vi "main_remote_old.vi"() -> ()   [LabVIEW 2019]
uses:
  Ctrl/SoutWork.ctl
  <vilib>/Utility/inputDevices.llb/keyboardAcquire.vi
  <vilib>/Utility/inputDevices.llb/closeKeyboard.vi
panel:
  in  "AGV status":string
  in  "buttton group":T1
  in  "tap":T2(tab)
  out "LiDAR Image Gray":T3(plugin-control)
  out "LiDAR Error":errorcluster
  out "Robot Status Error":errorcluster
  out "System Status Error":errorcluster
  out "Remote Control Command Error":errorcluster
  out "Vehicle Motion State Error":errorcluster
  in  "EStop Command":bool
  in  "Manual":bool
  in  "ChoosePath":u8
  in  "Stop AGV":bool
  in  "AGV Start":bool
  out "Error code high":bool[](array[boolean])
  out "Error code  low":bool[](array[boolean])
  out "Motor Over Current Alarm":bool
  out "Motor Over Current Protection":bool
  out "Motor Drive Over Temperature":bool
  out "System Status":T4
  out "Vehicle Motion State":T5
  out "robot status":T6
  out "Sensor Status":T7
  out "EStop Pressed":bool
  out "Image":T3(plugin-control)
  in  "OnboardPC IP":string="223.171.56.43"
  out "Index Y":dbl
  out "Index X":dbl
  out "Translational Vel (m/s)":dbl format="%4.2f"
  out "Rotational Vel (rad/s)":dbl format="%.2f"
  in  "stop":bool
  # "Mando GOLIE"
  # "Communication Error"
  # "<E-H>\nbit [0] Check error of CAN communication control command (0: No failure 1: Failure) \nbit [1] Motor drive over-temperature alarm[1] (0: No alarm 1: Alarm) Temperature limited to 55℃ \nbit [2] Motor over-current alarm[1] (0: No alarm 1: Alarm) Current effective value 15A \nbit [3] Battery under-voltage alarm (0: No alarm 1: Alarm) Alarm voltage 22.5V \nbit [4] RC transmitter disconnection protection (0: Normal 1: RC transmitter disconnected) \n\n<E-L>\nbit [0] Battery under-voltage failure (0: No failure 1: Failure) Protective voltage 22V \nbit [1] Battery over-voltage failure (0: No failure 1: Failure)  \nbit [2] No.1 motor communication failure (0: No failure 1: Failure)  \nbit [3] No.2 motor communication failure (0: No failure 1: Failure)  \nbit [4] No.3 motor communication failure (0: No failure 1: Failure)  \nbit [5] No.4 motor communication failure (0: No failure 1: Failure)  \nbit [6] Motor drive over-temperature protection[2] (0: No protection 1: Protection) Temperature limited to 65℃ \nbit [7] Motor over-current protection[2] (0: No protection 1: Protection) Current effective value 20A"
  # "bit [0] Battery under-voltage failure (0: No failure 1: Failure) Protective voltage 22V \nbit [1] Battery over-voltage failure (0: No failure 1: Failure)  \nbit [2] No.1 motor communication failure (0: No failure 1: Failure)  \nbit [3] No.2 motor communication failure (0: No failure 1: Failure)  \nbit [4] No.3 motor communication failure (0: No failure 1: Failure)  \nbit [5] No.4 motor communication failure (0: No failure 1: Failure)  \nbit [6] Motor drive over-temperature protection[2] (0: No protection 1: Protection) Temperature limited to 65℃ \nbit [7] Motor over-current protection[2] (0: No protection 1: Protection) Current effective value 20A"
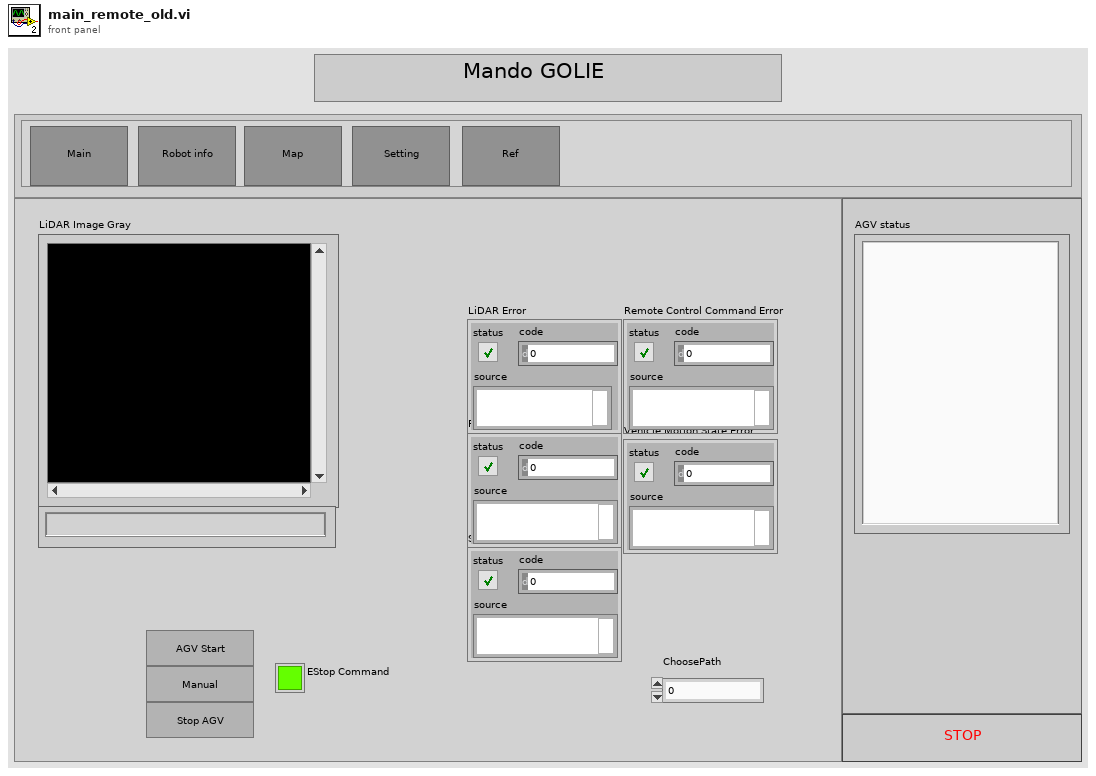
[diagram p1: front panel]
types:
  T1 = cluster{"Main":bool, "Main 2":bool, "Main 3":bool, "Main 4":bool, "Main 5":bool}
  T2 = enum32{"Main", "Robot info", "Map", "Setting", "Ref"}
  T3 = typedef "IMAQ Image.ctl" = refnum<image>
  T4 = cluster{"System Feedback":cluster{"system state":string, "Control Mode":u8, "Battery Voltage (V)":dbl, "error code High":u8, "error code Low":u8}}
  T5 = typedef "SoutWork.ctl" = enum16{"wait", "Move", "ObstacleStop", "EStop", "Goal"}
  T6 = cluster{"X (m)":dbl, "Y (m)":dbl, "Z (m)":dbl, "Roll (degree)":dbl, "Pitch (degree)":dbl, "Heading (degree)":dbl, "Linear velocity (m/s)":dbl, "Angular velocity (rad/s)":dbl}
  T7 = cluster{"VLP16 Sensor Error ":bool, "SICK Sensor Error":bool, "GNSS Sensor Error":bool, "Heading=0 Alarm":bool, "Obstacle Stop Alarm":bool}
  T8 = typedef "Image Type" = u32
  T9 = enum16{"0", "1", "2", "3", "4", "5", "6", "7", "8", "9", "A", "B", "C", "D", "E", "F", "G", "H", "I", "J", "K", "L", "M", "N", "O", "P", "Q", "R", "S", "T", "U", "V", "W", "X", "Y", "Z", "F1", "F2", "F3", "F4", "F5", "F6", "F7", "F8", "F9", "F10", "F11", "F12", "F13", "F14", "F15", "ADD", "BACK", "BACKSLASH", "CAPITAL", "COMMA", "DECIMAL", "DELETE", "DIVIDE", "DOWN", "END", "EQUALS", "ESCAPE", "GRAVE (`)", "HOME", "INSERT", "LBRACKET", "LCONTROL", "LEFT", "L ALT", "LSHIFT", "LWIN", "MINUS", "MULTIPLY", "NEXT", "NUMLOCK", "NUMPAD_0", "NUMPAD_1", "NUMPAD_2", "NUMPAD_3", "NUMPAD_4", "NUMPAD_5", "NUMPAD_6", "NUMPAD_7", "NUMPAD_8", "NUMPAD_9", "PAUSE", "PERIOD", "PRIOR (PG UP)", "RBRACKET", "RCONTROL", "RETURN", "RIGHT", "R ALT", "RSHIFT", "RWIN", "SCROLL", "SEMICOLON", "SLASH", "SPACE", "SUBTRACT", "TAB", "UP", "ENTER (num pad)", "' (quote)"}[]
  T10 = enum16{"0", "1", "2", "3", "4", "5", "6", "7", "8", "9", "A", "B", "C", "D", "E", "F", "G", "H", "I", "J", "K", "L", "M", "N", "O", "P", "Q", "R", "S", "T", "U", "V", "W", "X", "Y", "Z", "F1", "F2", "F3", "F4", "F5", "F6", "F7", "F8", "F9", "F10", "F11", "F12", "F13", "F14", "F15", "ADD", "BACK", "BACKSLASH", "CAPITAL", "COMMA", "DECIMAL", "DELETE", "DIVIDE", "DOWN", "END", "EQUALS", "ESCAPE", "GRAVE (`)", "HOME", "INSERT", "LBRACKET", "LCONTROL", "LEFT", "L ALT", "LSHIFT", "LWIN", "MINUS", "MULTIPLY", "NEXT", "NUMLOCK", "NUMPAD_0", "NUMPAD_1", "NUMPAD_2", "NUMPAD_3", "NUMPAD_4", "NUMPAD_5", "NUMPAD_6", "NUMPAD_7", "NUMPAD_8", "NUMPAD_9", "PAUSE", "PERIOD", "PRIOR (PG UP)", "RBRACKET", "RCONTROL", "RETURN", "RIGHT", "R ALT", "RSHIFT", "RWIN", "SCROLL", "SEMICOLON", "SLASH", "SPACE", "SUBTRACT", "TAB", "UP", "ENTER (num pad)", "' (quote)"}
  T11 = cluster{"Vehicle Motion State":u8, "Index X":dbl, "Index Y":dbl, bool}
  T12 = cluster{"Boolean array[0]":bool, "Boolean array[1]":bool, "Boolean array[2]":bool, "Boolean array[3]":bool, "Boolean array[4]":bool}
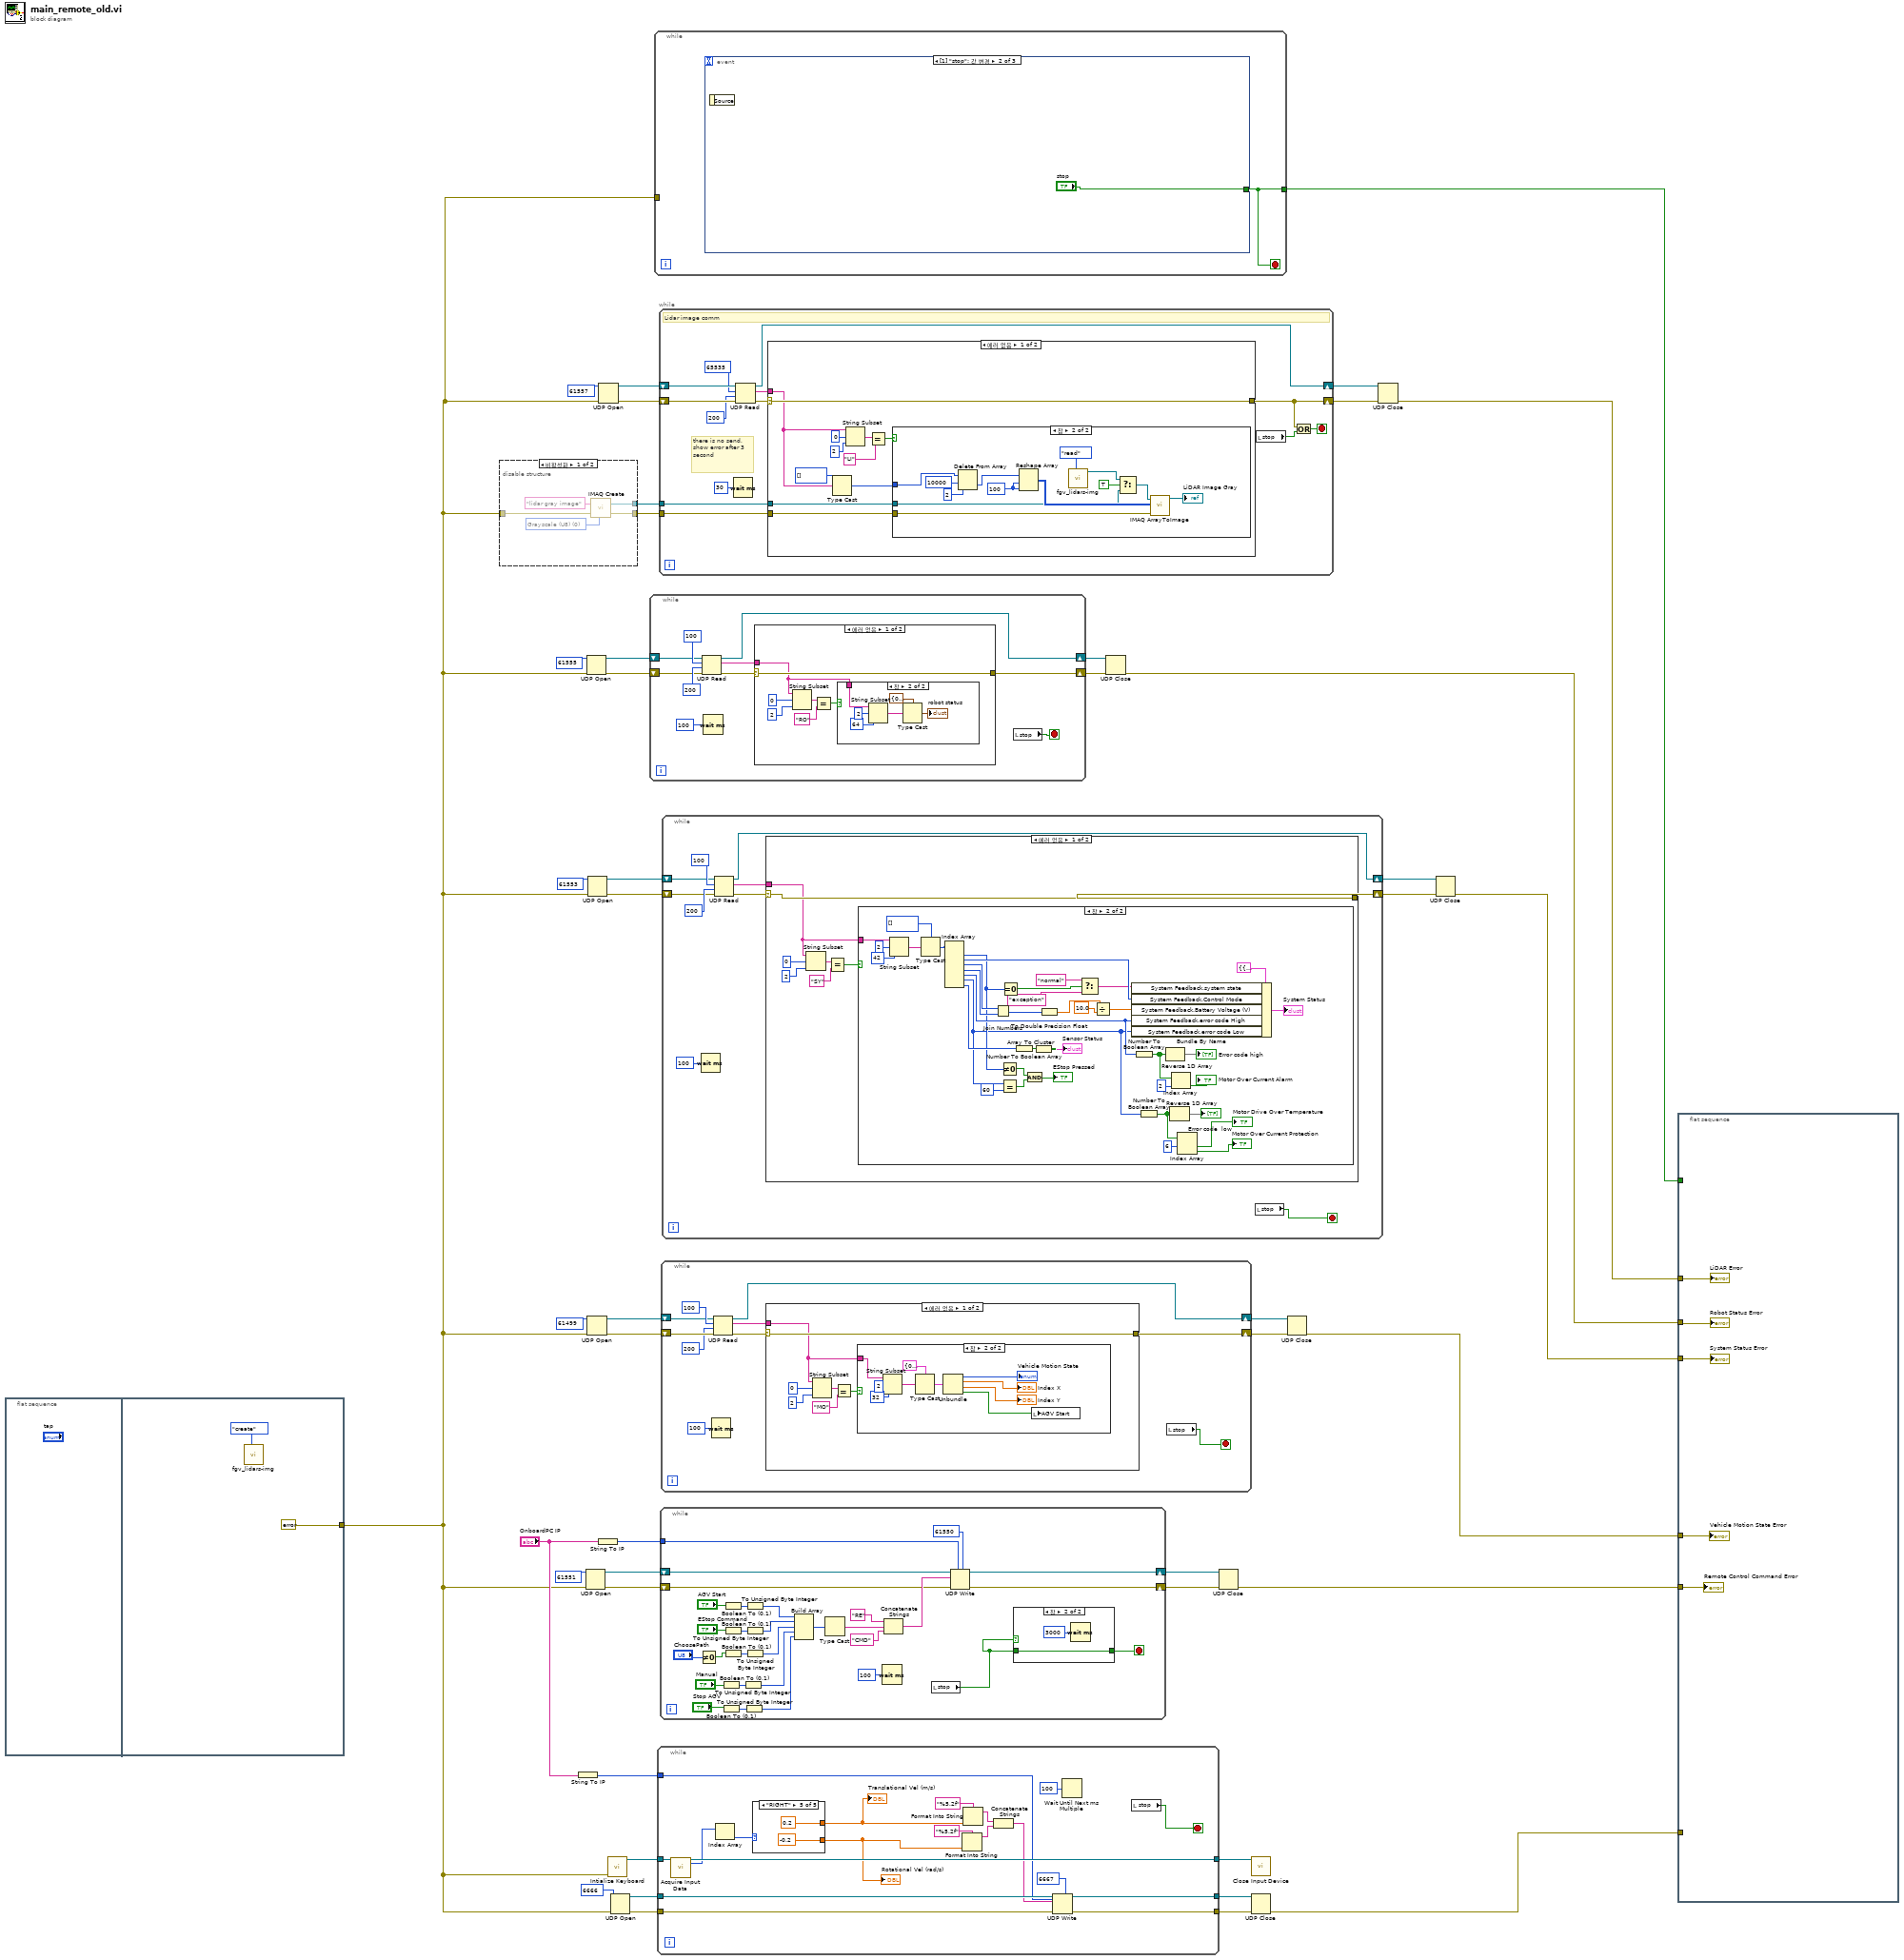
[diagram p0: block diagram]
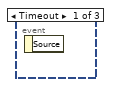
[diagram p3: hidden frame]
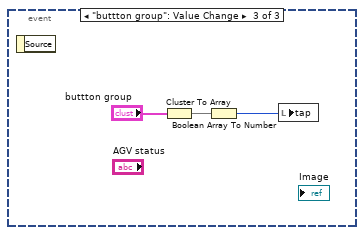
[diagram p4: hidden frame]
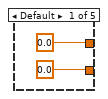
[diagram p5: hidden frame]
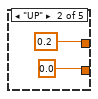
[diagram p6: hidden frame]
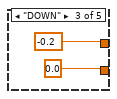
[diagram p7: hidden frame]
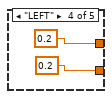
[diagram p8: hidden frame]
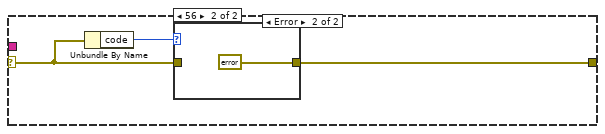
[diagram p10: hidden frame]
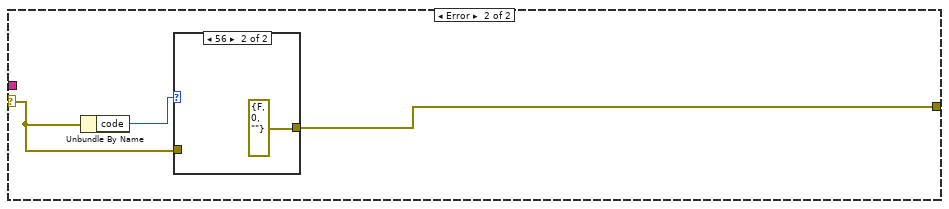
[diagram p14: hidden frame]
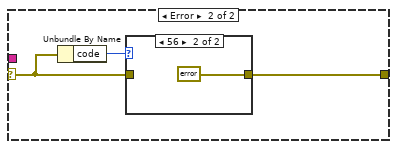
[diagram p17: hidden frame]
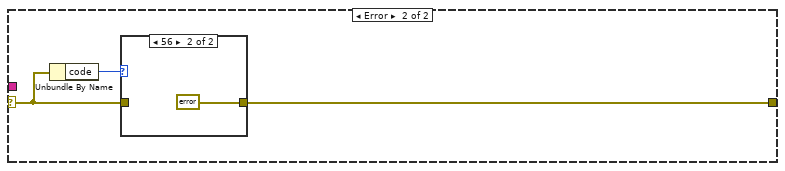
[diagram p20: hidden frame]
diagram:
  n1 = flat-sequence {
    tunnel: [errorcluster {"status"=FALSE, "code"=0, "source"=""} ("에러 입력(에러 없음)")] -> w8
    frame #0 {
    }
    frame #1 {
      n2 = call "fgv_lidars-img.vi"("cmd"=enum16{"create", "read", "close"}."create") -> ()  [unwired: 10 in, 1 out]
    }
  }
  n3 = disable-structure shown="비활성화" {
    disable-tunnel: [w50 _] -> w40
    disable-tunnel: [w49 _] -> w39
    disable-tunnel: w8 -> [w48 _]
    frame Disabled {
      w51 = T8 0 items=["Grayscale (U8)", "Grayscale (I16)", "Grayscale (SGL)", "Complex (CSG)", "RGB (U32)", "HSL (U32)", "RGB (U64)", "Grayscale (U16)"] ("Image Type")
      n4 = call "IMAQ Create"("Image Name"="lidar gray image", "Image Type"=w51, "error in (no error)"=w48) -> ("New Image"=w50:T3, "error out"=w49:errorcluster)  [unwired: 2 in]
    }
    frame Enabled {
    }
  }
  n5 = String To IP(1:"OnboardPC IP") -> (0:w9:u32)
  n6 = UDP Open(8:w8, 11:u16 61551 ("port")) -> (port=w27:refnum<k16>, 0:w26:errorcluster)  [unwired: 3 in, 1 out]
  n7 = UDP Open(8:w8, 11:u16 61555 ("port")) -> (port=w37:refnum<k16>, 0:w36:errorcluster)  [unwired: 3 in, 1 out]
  n8 = UDP Open(8:w8, 11:u16 61499 ("port")) -> (port=w21:refnum<k16>, 0:w20:errorcluster)  [unwired: 3 in, 1 out]
  n9 = UDP Open(8:w8, 11:u16 61553 ("port")) -> (port=w32:refnum<k16>, 0:w31:errorcluster)  [unwired: 3 in, 1 out]
  n10 = String To IP(1:"OnboardPC IP") -> (0:w23:u32)
  n11 = UDP Open(8:w8, 11:u16 61557 ("port")) -> (port=w45:refnum<k16>, 0:w44:errorcluster)  [unwired: 3 in, 1 out]
  n12 = call <vilib>:"Intialize Keyboard.vi"("error in (no error)"=w8) -> ("device ID"=w14:refnum<k1>)  [unwired: 9 in, 1 out]
  n13 = UDP Open(8:w8, 11:u16 6666 ("remote port or service name")) -> (port=w16:refnum<k16>, 0:w15:errorcluster)  [unwired: 3 in, 1 out]
  n14 = while {
    shift-right: [w56] -> w35
    shift-left: w37 -> [w60]
    shift-right: [w55] -> w34
    shift-left: w36 -> [w59]
    stop <- w53 stop-if-true
    n15 = UDP Read(connection ID=w60, max size (548)=100, timeout ms (25000)=200, 8:w59) -> (data out=w57:string, error out=w58:errorcluster, 3:w56:refnum<k16>)  [unwired: 2 out]
    n16 = Wait (ms)(milliseconds to wait=u32 100) -> ()  [unwired: 1 out]
    n17 = case shown="에러 없음" w58 {
      selector: w58 -> [w69 w77]
      tunnel: w57 -> [w63 _]
      tunnel: [w69 w76] -> w55
      frame No Error {
        n18 = String Subset(string=w63, offset (0)=0, length (rest)=2 ("length (rest)")) -> (substring=w66:string)
        n19 = Equal?(x=w66, y="RO") -> (x = y?=w64:bool)
        n20 = case shown="참" w64 {
          tunnel: w63 -> [_ w75]
          frame False {
          }
          frame True {
            n21 = String Subset(string=w75, offset (0)=2, length (rest)=64 ("length (rest)")) -> (substring=w71:string)
            n22 = Type Cast(type=T6 {"X (m)"=0.0, "Y (m)"=0.0, "Z (m)"=0.0, "Roll (degree)"=0.0, "Pitch (degree)"=0.0, "Heading (degree)"=0.0, "Linear velocity (m/s)"=0.0, "Angular velocity (rad/s)"=0.0} ("Robot Status"), x=w71) -> (*(type *) &x=→"robot status":T6)
          }
        }
      }
      frame Error {
        n23 = Unbundle By Name(w77) -> ("code"=w78:i32)
        n24 = case shown="56" w78 {
          tunnel: w77 -> [w79 _]
          tunnel: [w79 errorcluster {"status"=FALSE, "code"=0, "source"=""} ("error IO")] -> w76
          frame 0, Default {
          }
          frame 56 {
          }
        }
      }
    }
    n25 = local read "stop"() -> (w53:bool)
  }
  n26 = while {
    tunnel: w8 -> [_]
    tunnel: [w81] -> w1
    stop <- w81 stop-if-true
    n27 = event shown="[1] \"stop\": 값 변경" {
      selector: _ -> [_ _ _]
      dyn-events: _ -> [_ _ _]
      timeout: _ -> [_ _ _]
      tunnel: [_ "stop" _] -> w81
      event Timeout {
        n28 = event-data() -> ()  [unwired: 1 in, 1 out]
      }
      event "stop": Value Change {
        n29 = event-data() -> ()  [unwired: 1 in, 1 out]
      }
      event "buttton group": Value Change {
        n30 = event-data() -> ()  [unwired: 1 in, 1 out]
        n31 = Cluster To Array(cluster="buttton group") -> (array=w84:bool[])
        n32 = Boolean Array To Number(Boolean array=w84) -> (number=w83:u32)
        n33 = local write "tap"(w83) -> ()
      }
    }
  }
  n34 = while {
    tunnel: w14 -> [w104]
    tunnel: [w103] -> w17
    tunnel: w16 -> [w102]
    tunnel: [w101] -> w13
    tunnel: [w95] -> w12
    tunnel: w15 -> [w94]
    tunnel: w9 -> [w88]
    stop <- w86 stop-if-true
    # "Main Loop"
    n35 = call-poly <vilib>:"Acquire Input Data.vi"("device ID"=w104) -> ("device ID"=w103:refnum<k1>, "keys pressed"=w92:T9)  [unwired: 16 in, 1 out]
    n36 = Index Array(array=w92) -> (element=w91:T10)  [unwired: 1 in]
    n37 = case shown="\"RIGHT\"" w91 {
      tunnel: [0.0 ("Rotational Vel (rad/s)") 0.2 ("Rotational Vel (rad/s)") -0.2 ("Rotational Vel (rad/s)") 0.2 ("Rotational Vel (rad/s)") 0.2 ("Rotational Vel (rad/s)")] -> w90
      tunnel: [0.0 ("Rotational Vel (rad/s)") 0.0 ("Rotational Vel (rad/s)") 0.0 ("Rotational Vel (rad/s)") 0.2 ("Rotational Vel (rad/s)") -0.2 ("Rotational Vel (rad/s)")] -> w89
      frame Default {
      }
      frame "UP" {
      }
      frame "DOWN" {
      }
      frame "LEFT" {
      }
      frame "RIGHT" {
      }
    }
    "Translational Vel (m/s)" <- w90
    "Rotational Vel (rad/s)" <- w89
    n38 = Format Into String(format string="%5.2f", w89) -> (resulting string=w97:string)  [unwired: 2 in, 1 out]
    n39 = Format Into String(format string="%5.2f", w90) -> (resulting string=w98:string)  [unwired: 2 in, 1 out]
    n40 = Concatenate Strings(w98, w97) -> (w96:string)
    n41 = UDP Write(address=w88, port or service name=u16 6667, connection ID=w102, data in=w96, 8:w94) -> (error out=w95:errorcluster, 3:w101:refnum<k16>)  [unwired: 1 in]
    n42 = Wait Until Next ms Multiple(millisecond multiple=u32 100) -> ()  [unwired: 1 out]
    n43 = local read "stop"() -> (w86:bool)
  }
  n44 = while {
    shift-right: [w120] -> w43
    shift-left: w45 -> [w127]
    shift-right: [w119] -> w42
    shift-left: w44 -> [w126]
    tunnel: w40 -> [w118]
    tunnel: w39 -> [w117]
    stop <- w123 stop-if-true
    # "there is no send, show error after 3 second"
    # "Lidar image comm"
    n45 = Wait (ms)(milliseconds to wait=u32 30) -> ()  [unwired: 1 out]
    n46 = UDP Read(connection ID=w127, max size (548)=65535, timeout ms (25000)=200, 8:w126) -> (data out=w125:string, error out=w121:errorcluster, 3:w120:refnum<k16>)  [unwired: 2 out]
    n47 = case shown="에러 없음" w121 {
      selector: w121 -> [w137 w154]
      tunnel: w125 -> [w130 _]
      tunnel: [w137 w152] -> w119
      tunnel: w118 -> [w136 _]
      tunnel: w117 -> [w135 _]
      frame No Error {
        n48 = Type Cast(type=u8[] [], x=w130) -> (*(type *) &x=w128:u8[])
        n49 = String Subset(string=w130, offset (0)=0, length (rest)=2 ("length (rest)")) -> (substring=w132:string)
        n50 = Equal?(x=w132, y="LI") -> (x = y?=w129:bool)
        n51 = case shown="참" w129 {
          tunnel: w128 -> [_ w151]
          tunnel: w136 -> [_ w142]
          tunnel: w135 -> [_ w147]
          frame False {
          }
          frame True {
            w149 = 100 ("dimension size")
            n52 = Delete From Array(array=w151, length=10000, index=2) -> (deleted portion=w144:u8[])  [unwired: 1 out]
            n53 = Reshape Array(w144, w149, w149) -> (w148:u8[][])
            n54 = call "fgv_lidars-img.vi"("cmd"=enum16{"create", "read", "close"}."read") -> ("New Image"=w140:T3)  [unwired: 10 in]
            n55 = Select(t=w140, s=TRUE, f=w142) -> (s? t:f=w141:T3)
            n56 = call "IMAQ ArrayToImage"("error in (no error)"=w147, "Image Pixels (U8)"=w148, "Image"=w141) -> ("Image Out"=→"LiDAR Image Gray":T3)  [unwired: 7 in, 1 out]
          }
        }
      }
      frame Error {
        n57 = Unbundle By Name(w154) -> ("code"=w153:i32)
        n58 = case shown="56" w153 {
          tunnel: w154 -> [w155 _]
          tunnel: [w155 errorcluster {"status"=FALSE, "code"=0, "source"=""} ("error IO")] -> w152
          frame 0, Default {
          }
          frame 56 {
          }
        }
      }
    }
    n59 = local read "stop"() -> (w115:bool)
    n60 = Or(x=w119, y=w115) -> (x .or. y?=w123:bool)
  }
  n61 = while {
    shift-right: [w177] -> w25
    shift-left: w27 -> [w179]
    shift-right: [w176] -> w24
    shift-left: w26 -> [w178]
    tunnel: w23 -> [w180]
    stop <- w160 stop-if-true
    n62 = Not Equal To 0?(x="ChoosePath") -> (x != 0?=w159:bool)
    n63 = Boolean To (0,1)(Boolean="Manual") -> (0, 1=w166:i16)
    n64 = Boolean To (0,1)(Boolean="Stop AGV") -> (0, 1=w164:i16)
    n65 = Boolean To (0,1)(Boolean="AGV Start") -> (0, 1=w174:i16)
    n66 = Boolean To (0,1)(Boolean="EStop Command") -> (0, 1=w173:i16)
    n67 = Boolean To (0,1)(Boolean=w159) -> (0, 1=w169:i16)
    n68 = To Unsigned Byte Integer(number=w166) -> (unsigned 8bit integer=w165:u8)
    n69 = To Unsigned Byte Integer(number=w164) -> (unsigned 8bit integer=w162:u8)
    n70 = To Unsigned Byte Integer(number=w174) -> (unsigned 8bit integer=w172:u8)
    n71 = To Unsigned Byte Integer(number=w173) -> (unsigned 8bit integer=w171:u8)
    n72 = To Unsigned Byte Integer(number=w169) -> (unsigned 8bit integer=w168:u8)
    n73 = Build Array(w172, w171, w168, w165, w162) -> (w170:u8[])
    n74 = Type Cast(x=w170) -> (*(type *) &x=w184:string)  [unwired: 1 in]
    n75 = Wait (ms)(milliseconds to wait=u32 100) -> ()  [unwired: 1 out]
    n76 = Concatenate Strings("RE", w184, "CMD" ("string")) -> (w185:string)
    n77 = local read "stop"() -> (w157:bool)
    n78 = UDP Write(address=w180, port or service name=u16 61550, connection ID=w179, data in=w185, 8:w178) -> (error out=w176:errorcluster, 3:w177:refnum<k16>)  [unwired: 1 in]
    n79 = case shown="참" w157 {
      tunnel: [w187 w189] -> w160
      tunnel: w157 -> [w187 w189]
      frame False {
      }
      frame True {
        n80 = Wait (ms)(milliseconds to wait=u32 3000) -> ()  [unwired: 1 out]
      }
    }
  }
  n81 = while {
    shift-right: [w194] -> w19
    shift-left: w21 -> [w198]
    shift-right: [w193] -> w18
    shift-left: w20 -> [w197]
    stop <- w190 stop-if-true
    n82 = Wait (ms)(milliseconds to wait=u32 100) -> ()  [unwired: 1 out]
    n83 = UDP Read(connection ID=w198, max size (548)=100, timeout ms (25000)=200, 8:w197) -> (data out=w195:string, error out=w196:errorcluster, 3:w194:refnum<k16>)  [unwired: 2 out]
    n84 = case shown="에러 없음" w196 {
      selector: w196 -> [w206 w218]
      tunnel: w195 -> [w200 _]
      tunnel: [w206 w217] -> w193
      frame No Error {
        n85 = String Subset(string=w200, offset (0)=0, length (rest)=2 ("length (rest)")) -> (substring=w203:string)
        n86 = Equal?(x=w203, y="MO") -> (x = y?=w201:bool)
        n87 = case shown="참" w201 {
          tunnel: w200 -> [_ w216]
          frame False {
          }
          frame True {
            n88 = String Subset(string=w216, offset (0)=2, length (rest)=32 ("length (rest)")) -> (substring=w213:string)
            n89 = Type Cast(type=T11 {"Vehicle Motion State"=0, "Index X"=0.0, "Index Y"=0.0, FALSE}, x=w213) -> (*(type *) &x=w212:T11)
            n90 = Unbundle(w212) -> ("Vehicle Motion State"=→"Vehicle Motion State":u8, "Index X"=→"Index X":dbl, "Index Y"=→"Index Y":dbl, w207:bool)
            n91 = local write "AGV Start"(w207) -> ()
          }
        }
      }
      frame Error {
        n92 = Unbundle By Name(w218) -> ("code"=w219:i32)
        n93 = case shown="56" w219 {
          tunnel: w218 -> [w220 _]
          tunnel: [w220 errorcluster {"status"=FALSE, "code"=0, "source"=""} ("error IO")] -> w217
          frame 0, Default {
          }
          frame 56 {
          }
        }
      }
    }
    n94 = local read "stop"() -> (w190:bool)
  }
  n95 = while {
    shift-right: [w225] -> w30
    shift-left: w32 -> [w229]
    shift-right: [w224] -> w29
    shift-left: w31 -> [w228]
    stop <- w222 stop-if-true
    n96 = Wait (ms)(milliseconds to wait=u32 100) -> ()  [unwired: 1 out]
    n97 = UDP Read(connection ID=w229, max size (548)=100, timeout ms (25000)=200, 8:w228) -> (data out=w226:string, error out=w227:errorcluster, 3:w225:refnum<k16>)  [unwired: 2 out]
    n98 = case shown="에러 없음" w227 {
      selector: w227 -> [w238 w278]
      tunnel: w226 -> [w232 _]
      tunnel: [w238 w277] -> w224
      frame No Error {
        n99 = String Subset(string=w232, offset (0)=0, length (rest)=2 ("length (rest)")) -> (substring=w235:string)
        n100 = Equal?(x=w235, y="SY") -> (x = y?=w233:bool)
        n101 = case shown="참" w233 {
          tunnel: w232 -> [_ w276]
          frame False {
          }
          frame True {
            n102 = String Subset(string=w276, offset (0)=2, length (rest)=42 ("length (rest)")) -> (substring=w273:string)
            n103 = Type Cast(type=u8[] [], x=w273) -> (*(type *) &x=w264:u8[])
            n104 = Index Array(array=w264) -> (element #1=w251:u8, element #2=w263:u8, element #3=w262:u8, element #4=w261:u8, element #5=w254:u8, element #6=w250:u8, element #7=w259:u8)  [unwired: 7 in]
            n105 = Join Numbers(hi=w262, lo=w261) -> ((hi.lo)=w270:u16)
            n106 = Not Equal To 0?(x=w251) -> (x != 0?=w248:bool)
            n107 = Equal?(x=w250, y=u8 60) -> (x = y?=w247:bool)
            n108 = Equal To 0?(x=w251) -> (x = 0?=w269:bool)
            n109 = Number To Boolean Array(number=w259) -> (Boolean array=w257:bool[])
            n110 = And(x=w248, y=w247) -> (x .and. y?=→"EStop Pressed":bool)
            n111 = Array To Cluster(array=w257) -> (cluster=→"Sensor Status":T12)
            n112 = To Double Precision Float(number=w270) -> (double precision float=w271:dbl)
            n113 = Select(t="normal", s=w269, f="exception") -> (s? t:f=w252:string)
            n114 = Divide(x=w271, y=10.0) -> (x/y=w272:dbl)
            n115 = Bundle By Name(cluster=T4 {"System Feedback"={"system state"="", "Control Mode"=0, "Battery Voltage (V)"=0.0, "error code High"=0, "error code Low"=0}} ("System Status"), "System Feedback.system state"=w252, "System Feedback.Control Mode"=w263, "System Feedback.Battery Voltage (V)"=w272, "System Feedback.error code High"=w254, "System Feedback.error code Low"=w250) -> (→"System Status":T4)
            n116 = Number To Boolean Array(number=w254) -> (Boolean array=w245:bool[])
            n117 = Number To Boolean Array(number=w250) -> (Boolean array=w241:bool[])
            n118 = Reverse 1D Array(array=w245) -> (reversed array=→"Error code high":bool[])
            n119 = Reverse 1D Array(array=w241) -> (reversed array=→"Error code  low":bool[])
            n120 = Index Array(array=w245, index=2) -> (element=→"Motor Over Current Alarm":bool)
            n121 = Index Array(array=w241, index #1=6 ("index")) -> (element #1=→"Motor Drive Over Temperature":bool, element #2=→"Motor Over Current Protection":bool)  [unwired: 1 in]
          }
        }
      }
      frame Error {
        n122 = Unbundle By Name(w278) -> ("code"=w279:i32)
        n123 = case shown="56" w279 {
          tunnel: w278 -> [w280 _]
          tunnel: [w280 errorcluster {"status"=FALSE, "code"=0, "source"=""} ("error IO")] -> w277
          frame 0, Default {
          }
          frame 56 {
          }
        }
      }
    }
    n124 = local read "stop"() -> (w222:bool)
  }
  n125 = UDP Close(connection ID=w35, 8:w34) -> (error out=w3:errorcluster)  [unwired: 1 out]
  n126 = UDP Close(connection ID=w25, 8:w24) -> (error out=w7:errorcluster)  [unwired: 1 out]
  n127 = call-poly <vilib>:"Close Input Device.vi"("device ID"=w17) -> ()  [unwired: 9 in, 1 out]
  n128 = UDP Close(connection ID=w13, 8:w12) -> (error out=w6:errorcluster)  [unwired: 1 out]
  n129 = UDP Close(connection ID=w19, 8:w18) -> (error out=w5:errorcluster)  [unwired: 1 out]
  n130 = UDP Close(connection ID=w43, 8:w42) -> (error out=w2:errorcluster)  [unwired: 1 out]
  n131 = UDP Close(connection ID=w30, 8:w29) -> (error out=w4:errorcluster)  [unwired: 1 out]
  n132 = flat-sequence {
    tunnel: w7 -> [w286]
    tunnel: w6 -> [_]
    tunnel: w5 -> [w285]
    tunnel: w4 -> [w284]
    tunnel: w3 -> [w283]
    tunnel: w2 -> [w282]
    tunnel: w1 -> [_]
    frame #0 {
      "Remote Control Command Error" <- w286
      "Vehicle Motion State Error" <- w285
      "System Status Error" <- w284
      "Robot Status Error" <- w283
      "LiDAR Error" <- w282
    }
  }
